vi "Convert CDB Wfm to TCP String.vi"(7 "Format (Intlvd I16)":enum16{"Interleaved I16", "Interleaved DBL"}(ring), 8 "error in (no error)":errorcluster, 11 "CDB Wfm in":waveform(cdb)) -> (0 "error out":errorcluster, 2 "Message size":string, 3 "TCP message":string, 4 "max value":i16)   [LabVIEW 2015, in "Monitoring_receiver.lvlib"]
uses:
  Monitoring_receiver.lvlib
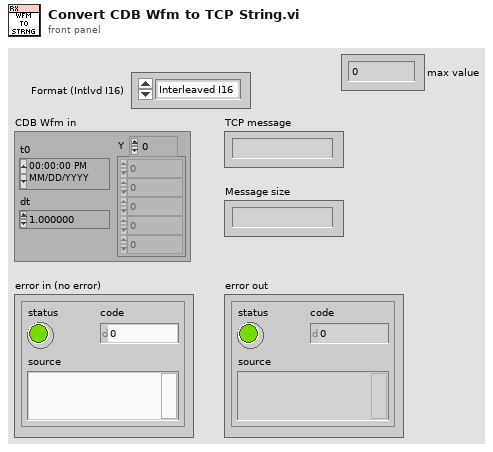
[diagram p1: front panel]
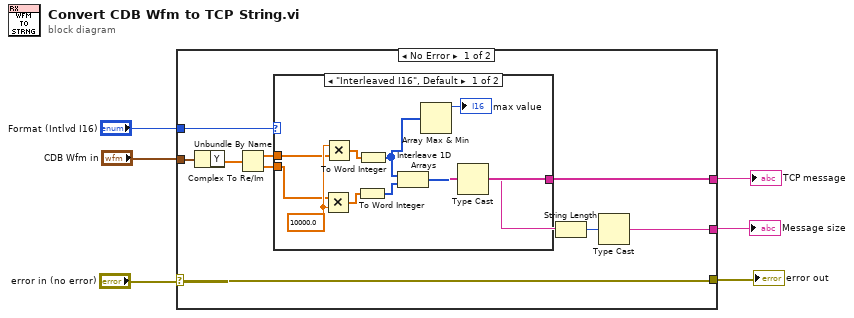
[diagram p0: block diagram]
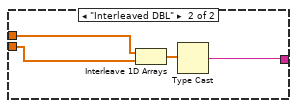
[diagram p2: hidden frame]
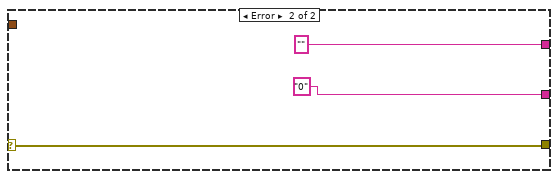
[diagram p3: hidden frame]
diagram:
  n1 = case shown="No Error" "error in (no error)" {
    selector: "error in (no error)" -> [w12 w32]
    tunnel: [w14 "0"] -> w2
    tunnel: [w13 ""] -> w3
    tunnel: "CDB Wfm in" -> [w11 _]
    tunnel: [w12 w32] -> w6
    tunnel: "Format (Intlvd I16)" -> [w7 _]
    frame No Error {
      n2 = Unbundle By Name(w11) -> ("Y"=w10:cdb[])
      n3 = Complex To Re/Im(x + iy=w10) -> (x=w9:dbl[], y=w8:dbl[])
      n4 = case shown="\"Interleaved I16\", Default" w7 {
        tunnel: [w25 w26] -> w13
        tunnel: w9 -> [w19 w29]
        tunnel: w8 -> [w18 w28]
        frame "Interleaved I16", Default {
          w20 = 10000.0
          n5 = Multiply(x=w18, y=w20) -> (x*y=w21:dbl[])
          n6 = Multiply(x=w20, y=w19) -> (x*y=w22:dbl[])
          n7 = To Word Integer(number=w21) -> (16bit integer=w23:i16[])
          n8 = To Word Integer(number=w22) -> (16bit integer=w17:i16[])
          n9 = Interleave 1D Arrays(w17, w23) -> (w24:i16[])
          n10 = Array Max & Min(array=w17) -> (max value=→"max value":i16)  [unwired: 3 out]
          n11 = Type Cast(x=w24) -> (*(type *) &x=w25:string)  [unwired: 1 out]
        }
        frame "Interleaved DBL" {
          n12 = Interleave 1D Arrays(w29, w28) -> (w27:dbl[])
          n13 = Type Cast(x=w27) -> (*(type *) &x=w26:string)  [unwired: 1 out]
        }
      }
      n14 = String Length(string=w13) -> (length=w15:i32)
      n15 = Type Cast(x=w15) -> (*(type *) &x=w14:string)  [unwired: 1 out]
    }
    frame Error {
    }
  }
  "error out" <- w6
  "TCP message" <- w3
  "Message size" <- w2
